vi "TDMS-File Viewer.vi"(4 "error in (no error)":errorcluster, 7 "file path":path) -> (0 "error out":errorcluster, 3 "file path out":path)   [LabVIEW 2010]
doc: "Opens the .tdms file specified in the <B>file path</B> input and presents the file data in the TDMS File Viewer dialog box."
uses:
  <vilib>/Utility/tdmsutil.llb/fileViewerConfigData.ctl
  <vilib>/Utility/tdmsutil.llb/TDMSFileViewerLocalizedText.vi
  Instance           1 26Saved   TDMS - File Viewer .vi
panel:
  in  "Help":bool
  in  "Status":string
  in  "Quit":bool
  in  "Settings...":bool
  in  "Properties / Values / Graph":T1(tab)
  in  "Properties":i32(listbox)
  in  "Raw data values":i32(listbox)
  out "Waveform Graph":waveform(dbl)[](graph)
  in  "File contents":string(tree)
  # "Displaying values 1..1000"
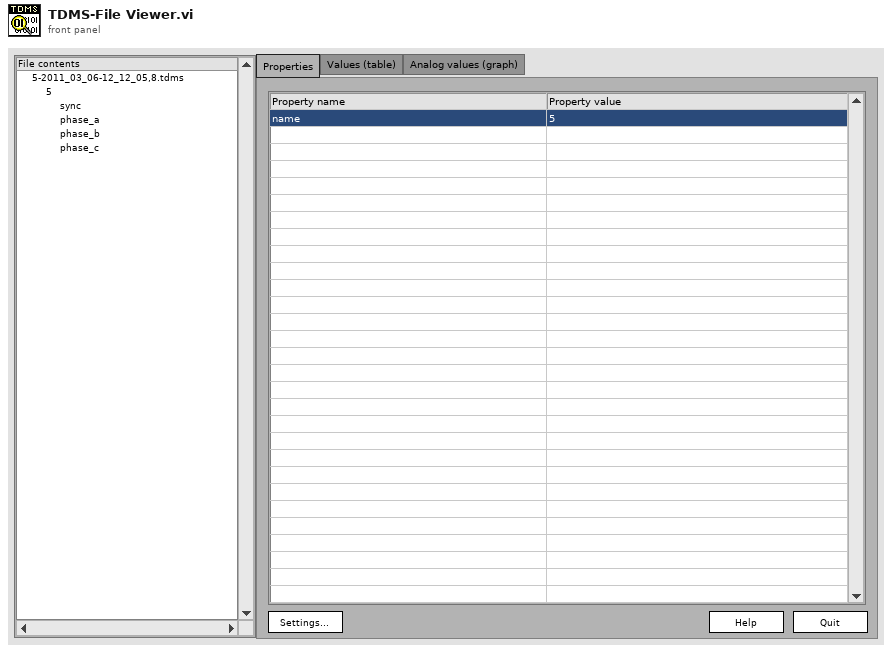
[diagram p1: front panel]
types:
  T1 = enum32{"Properties", "Values (table)", "Analog values (graph)"}
  T2 = enum16{"open", "open or create", "create or replace", "create", "open (read-only)"}
  T3 = typedef "fileViewerConfigData.ctl" = cluster{"Show all (table)":bool, "Show all (graph)":bool, "limit (table)":u64, "limit (graph)":u64, "no show":bool, "start (table)":u64, "start (graph)":u64}
  T4 = cluster{"Tree":refnum<vi>, "Tab Control":refnum<vi>, "property list":refnum<vi>, "raw data list":refnum<vi>, "Waveform Graph":refnum<vi>, "Ok":refnum<vi>, "Ok 2":refnum<vi>, "Ok 3":refnum<vi>, "Ok 4":refnum<vi>}
  T5 = typedef "LVRectTypeDef.ctl" = cluster{"left":i16, "top":i16, "right":i16, "bottom":i16}
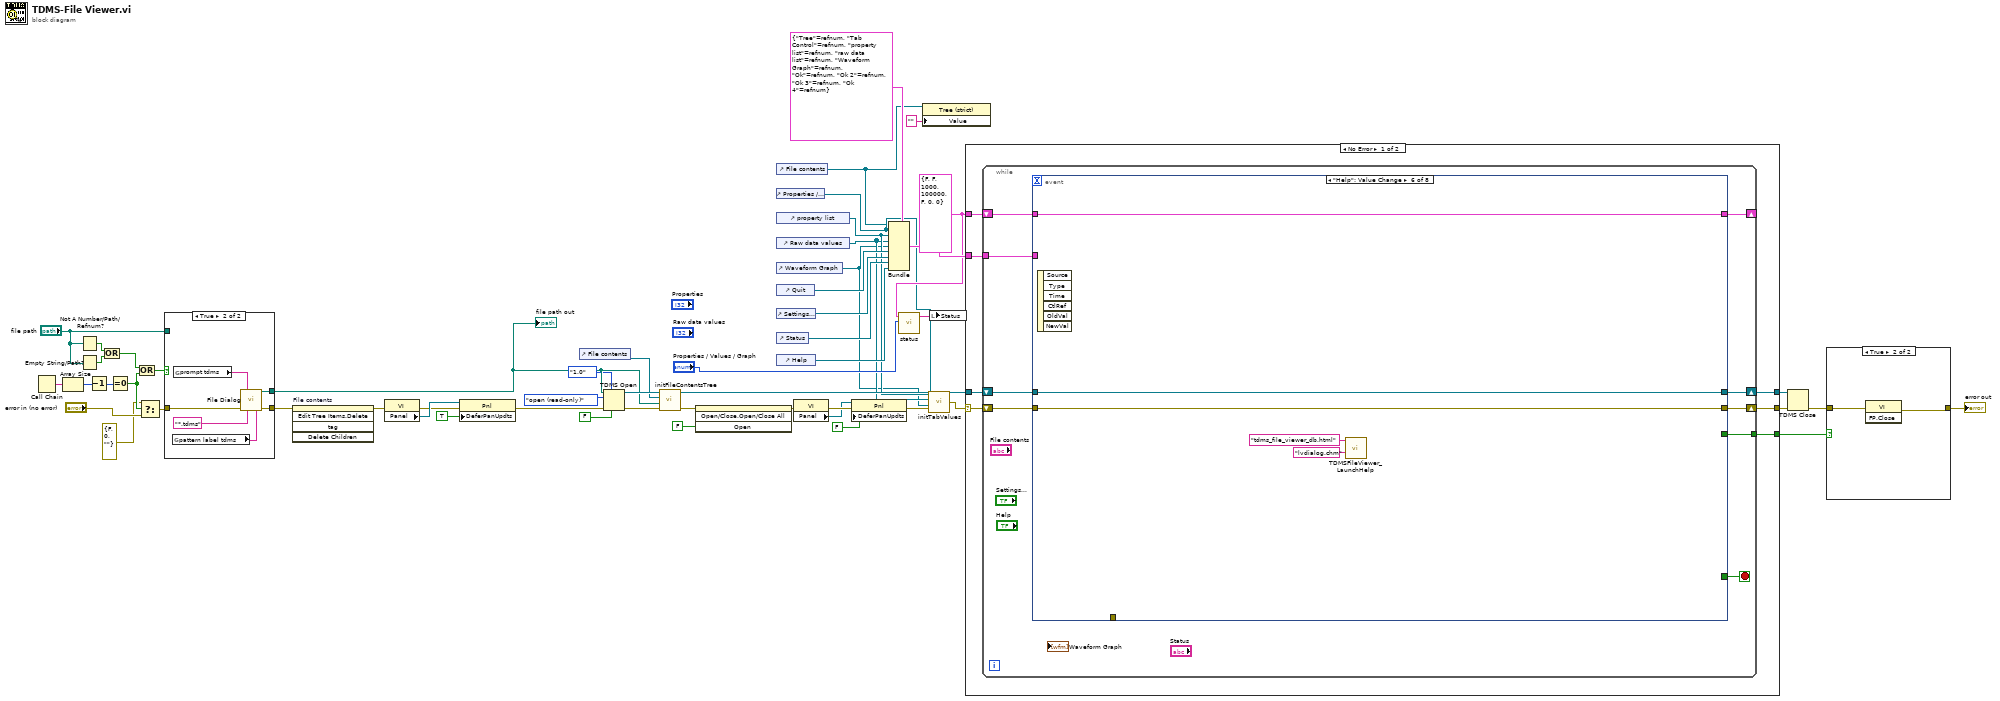
[diagram p0: block diagram]
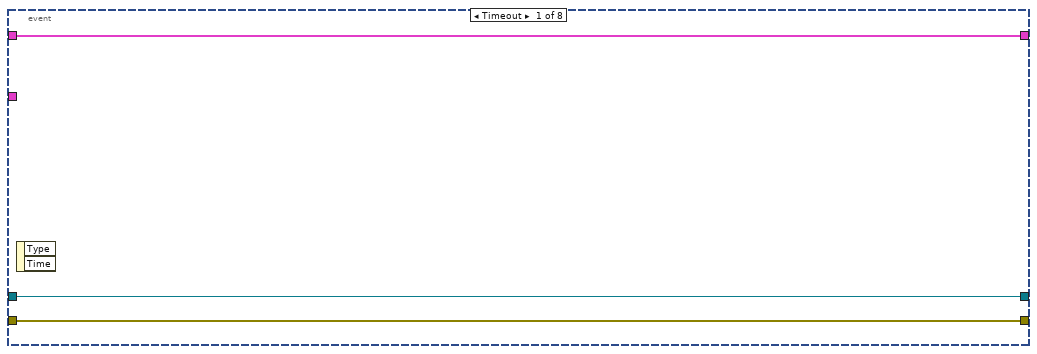
[diagram p3: hidden frame]
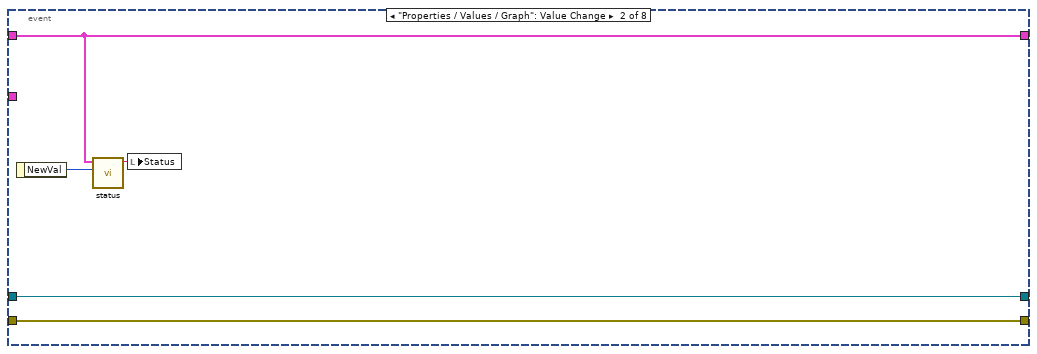
[diagram p4: hidden frame]
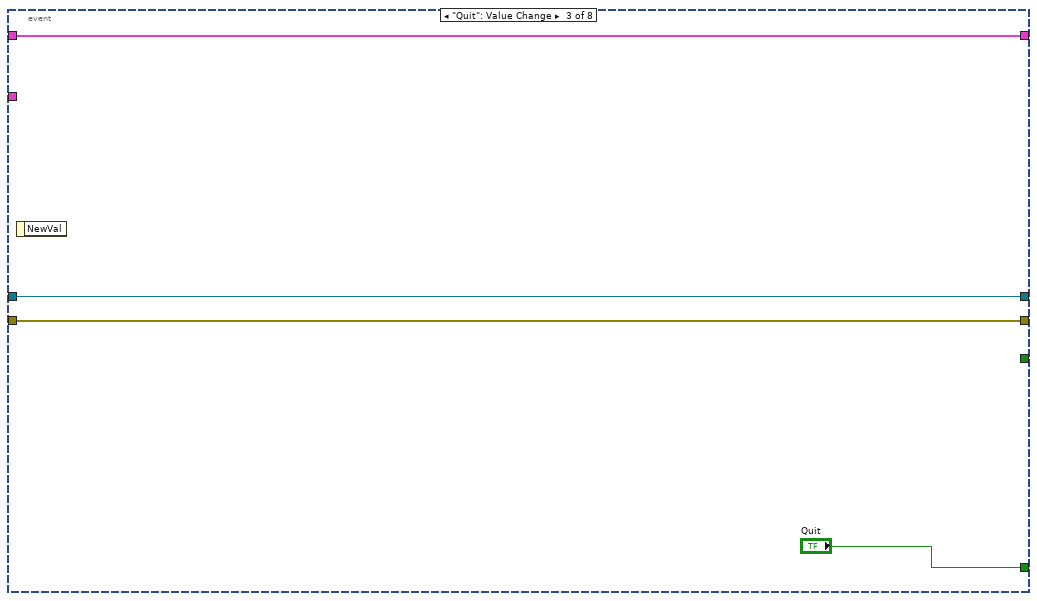
[diagram p5: hidden frame]
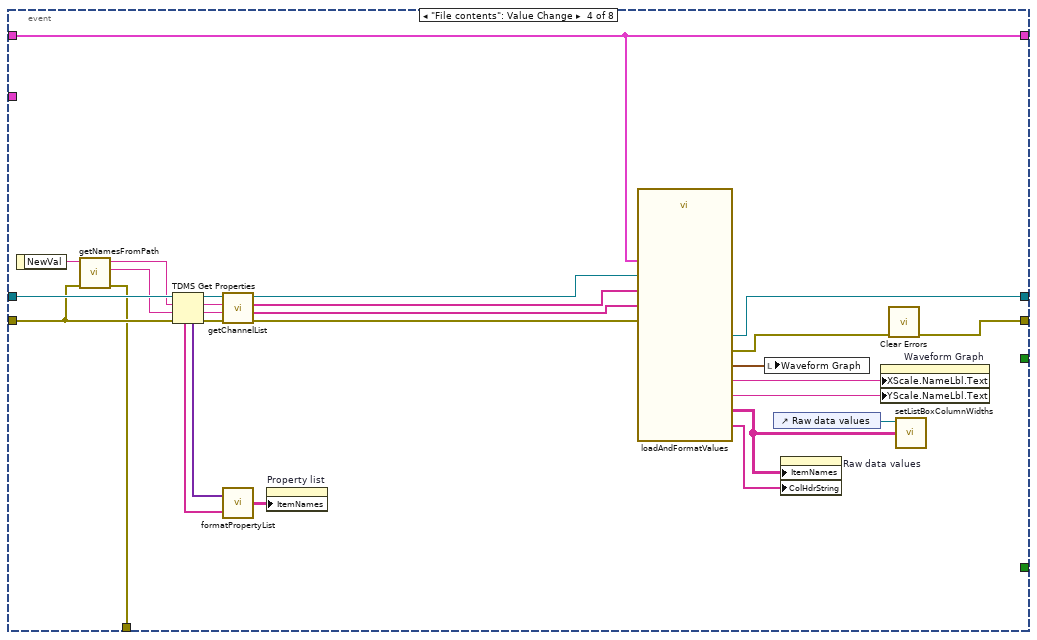
[diagram p6: hidden frame]
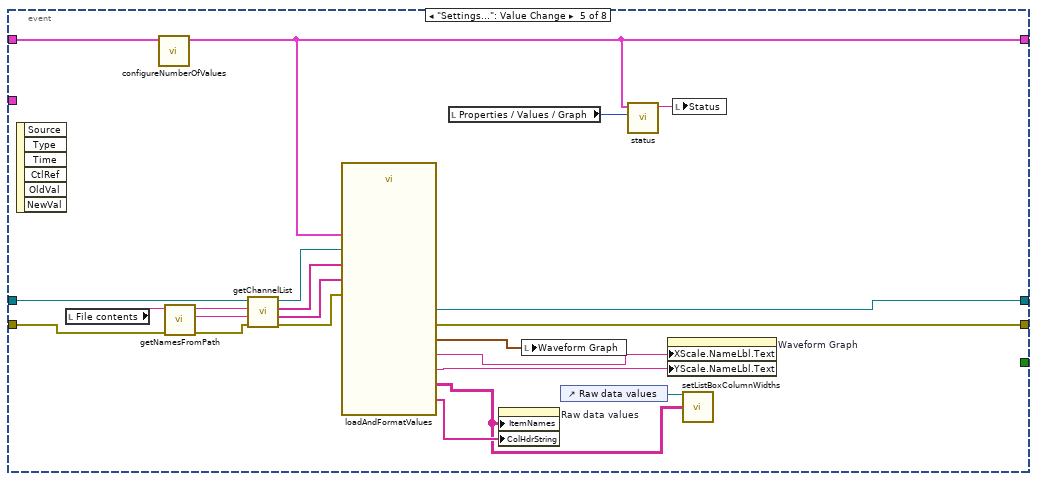
[diagram p7: hidden frame]
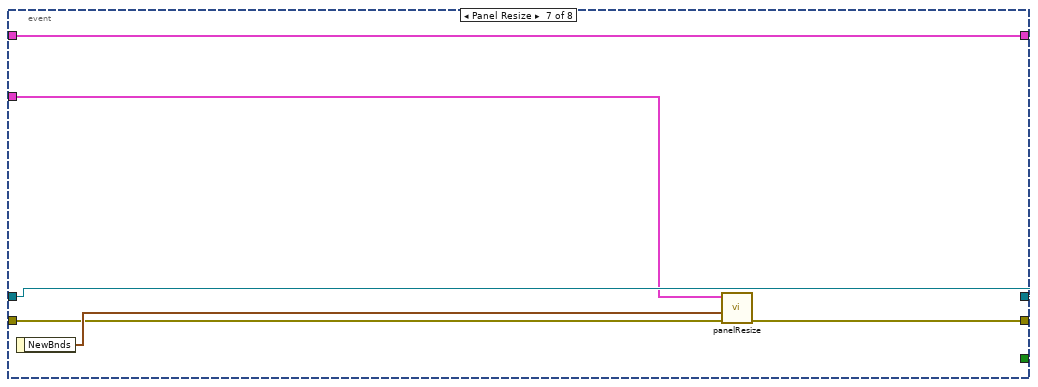
[diagram p8: hidden frame]
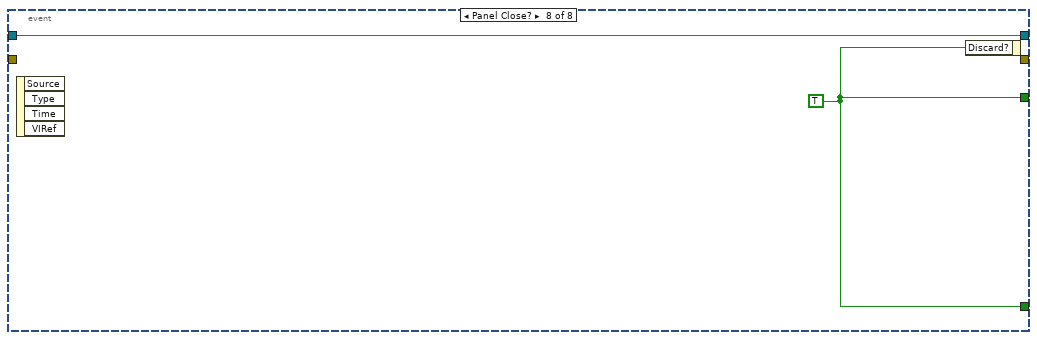
[diagram p9: hidden frame]
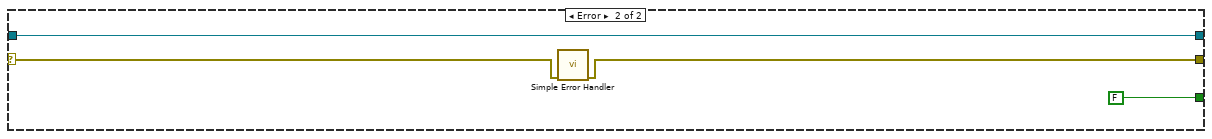
[diagram p10: hidden frame]
diagram:
  w20 = T3 {"Show all (table)"=FALSE, "Show all (graph)"=FALSE, "limit (table)"=1000, "limit (graph)"=100000, "no show"=FALSE, "start (table)"=0, "start (graph)"=0} ("TDMS File Viewer Configuration")
  n1 = Call Chain() -> (call chain=w35:string[])
  n2 = Array Size(array=w35) -> (size(s)=w33:i32)
  n3 = Not A Number/Path/Refnum?(number/path/refnum="file path") -> (NaN/Path/Refnum?=w37:bool)
  n4 = Empty String/Path?(string/path="file path") -> (empty?=w36:bool)
  n5 = Decrement(x=w33) -> (x-1=w32:i32)
  n6 = Or(x=w37, y=w36) -> (x .or. y?=w34:bool)
  n7 = Equal To 0?(x=w32) -> (x = 0?=w18:bool)
  n8 = Or(x=w34, y=w18) -> (x .or. y?=w31:bool)
  n9 = Select(t=errorcluster {"status"=FALSE, "code"=0, "source"=""}, s=w18, f="error in (no error)") -> (s? t:f=w17:errorcluster)
  n10 = case shown="True" w31 {
    tunnel: [w56 w62] -> w24
    tunnel: "file path" -> [w56 _]
    tunnel: [w55 w60] -> w23
    tunnel: w17 -> [w55 w59]
    frame False {
    }
    frame True {
      n11 = global read "TDMSFileViewerLocalizedText.vi" "pattern label tdms"() -> (w57:string)
      n12 = global read "TDMSFileViewerLocalizedText.vi" "prompt tdms"() -> (w58:string)
      n13 = call "File Dialog"("prompt"=w58, "error in"=w59, "pattern (all files)"="*.tdms", "pattern label"=w57) -> ("selected path"=w62:path, "error out"=w60:errorcluster)  [unwired: 3 in, 7 out]
    }
  }
  "file path out" <- w24
  n14 = invoke on="File contents" class="Tree (strict)" method="Edit Tree Items.Delete"(error in=w23) -> (error out=w45:errorcluster)  [unwired: 4 in, 4 out]
  n15 = property class="VI"(error in=w45) -> (error out=w46:errorcluster, "Panel"=w47:refnum<vi>)  [unwired: 1 in, 1 out]
  n16 = property class="Pnl"(reference=w47, error in=w46, "DeferPanUpdts"=TRUE ("Defer Panel Updates")) -> (error out=w49:errorcluster)  [unwired: 1 out]
  n17 = control-ref of="File contents"() -> (w25:refnum<vi>)
  n18 = TDMS Open(6:FALSE ("disable buffering (T)"), 7:enum16{"1.0", "2.0"}."1.0" ("file format version (2.0)"), 8:w49, 10:T2."open (read-only)" ("operation"), 11:w24) -> (0:w54:errorcluster, 3:w53:refnum<k34>)  [unwired: 1 in]
  n19 = call <vilib>:"initFileContentsTree.vi"("error in (no error)"=w54, "file path"=w24, "Tree Refnum"=w25, "tdms file"=w53) -> ("error out"=w41:errorcluster, "tdms file out"=w52:refnum<k34>)  [unwired: 2 out]
  n20 = invoke on="File contents" class="Tree (strict)" method="Open/Close.Open/Close All"(error in=w41, "Open"=FALSE ("Open?")) -> (error out=w40:errorcluster)  [unwired: 2 in, 3 out]
  n21 = control-ref of="File contents"() -> (w2:refnum<vi>)
  n22 = control-ref of="Properties / Values / Graph"() -> (w3:refnum<vi>)
  n23 = control-ref of="property list"() -> (w6:refnum<vi>)
  n24 = control-ref of="Raw data values"() -> (w5:refnum<vi>)
  n25 = control-ref of="Waveform Graph"() -> (w4:refnum<vi>)
  n26 = control-ref of="Quit"() -> (w29:refnum<vi>)
  n27 = control-ref of="Settings..."() -> (w27:refnum<vi>)
  n28 = control-ref of="Status"() -> (w22:refnum<vi>)
  n29 = control-ref of="Help"() -> (w9:refnum<vi>)
  n30 = property class="VI"(error in=w40) -> (error out=w43:errorcluster, "Panel"=w42:refnum<vi>)  [unwired: 1 in, 1 out]
  n31 = property class="Pnl"(reference=w42, error in=w43, "DeferPanUpdts"=FALSE ("Defer Panel Updates")) -> (error out=w8:errorcluster)  [unwired: 1 out]
  n32 = Bundle(cluster=T4 {"Tree"=refnum, "Tab Control"=refnum, "property list"=refnum, "raw data list"=refnum, "Waveform Graph"=refnum, "Ok"=refnum, "Ok 2"=refnum, "Ok 3"=refnum, "Ok 4"=refnum} ("control refs"), "Tree"=w2, "Tab Control"=w3, "property list"=w6, "raw data list"=w5, "Waveform Graph"=w4, "Ok"=w29, "Ok 2"=w27, "Ok 3"=w22, "Ok 4"=w9) -> (w30:T4)
  n33 = call <vilib>:"status.vi"("tab sheet"="Properties / Values / Graph", "TDMS File Viewer Configuration"=w20) -> ("status"=w21:string)  [unwired: 5 out]
  n34 = property class="Tree (strict)"(reference=w2, "Value"="") -> ()  [unwired: 1 in, 2 out]
  n35 = call <vilib>:"initTabValues.vi"("properties"=w6, "Values"=w5, "waveform"=w4, "error in"=w8, "Properties / Values / Graph"=w3) -> ("error out"=w7:errorcluster)
  n36 = local write "Status"(w21) -> ()
  n37 = case shown="No Error" w7 {
    selector: w7 -> [w64 w155]
    tunnel: w52 -> [w69 w156]
    tunnel: [w68 w156] -> w51
    tunnel: [w67 w154] -> w50
    tunnel: w30 -> [w66 _]
    tunnel: w20 -> [w65 _]
    tunnel: [w63 FALSE] -> w14
    frame No Error {
      n38 = while {
        shift-right: [w76] -> w67
        shift-left: w64 -> [w77]
        shift-right: [w75] -> w68
        shift-left: w69 -> [w78]
        tunnel: w66 -> [w73]
        shift-right: [w71] -> _
        shift-left: w65 -> [w72]
        tunnel: [w70] -> w63
        stop <- w74 stop-if-true
        n39 = event shown="[5] \"Help\": Value Change" {
          selector: _ -> [_ _ _ _ _ _ _ _]
          dyn-events: _ -> [_ _ _ _ _ _ _ _]
          timeout: _ -> [_ _ _ _ _ _ _ _]
          tunnel: w78 -> [w80 w85 w89 w117 w128 w143 w150 w152]
          tunnel: w77 -> [w81 w86 w88 w109 w136 w142 w147 _]
          tunnel: [w81 w86 w88 w104 w137 w142 w146 _] -> w76
          tunnel: [w80 w85 w89 w116 w138 w143 w150 w152] -> w75
          tunnel: [_ _ "Quit" _ _ _ _ w151] -> w74
          tunnel: [_ _ _ w108 _ _ _ _] -> _
          tunnel: w73 -> [_ _ _ _ _ _ w148 _]
          tunnel: w72 -> [w79 w82 w87 w97 w139 w144 w145 _]
          tunnel: [w79 w82 w87 w97 w118 w144 w145 _] -> w71
          tunnel: [_ _ _ _ _ _ _ w151] -> w70
          event Timeout {
            n40 = event-data() -> ()  [unwired: 3 out]
          }
          event "Properties / Values / Graph": Value Change {
            n41 = event-data() -> ("NewVal"=w84:T1)  [unwired: 1 out]
            n42 = call <vilib>:"status.vi"("tab sheet"=w84, "TDMS File Viewer Configuration"=w82) -> ("status"=w83:string)  [unwired: 5 out]
            n43 = local write "Status"(w83) -> ()
          }
          event "Quit": Value Change {
            n44 = event-data() -> ()  [unwired: 2 out]
          }
          event "File contents": Value Change {
            n45 = event-data() -> ("NewVal"=w111:string)  [unwired: 1 out]
            n46 = call <vilib>:"getNamesFromPath.vi"("error in (no error)"=w109, "tree path"=w111) -> ("error out"=w108:errorcluster, "channel"=w114:string, "group"=w115:string)  [unwired: 3 out]
            n47 = TDMS Get Properties(8:w109, 9:w114, 10:w115, 11:w117) -> (0:w102:errorcluster, 1:w101:string, 2:w95:string, 3:w103:refnum<k34>, 4:w112:variant[], 6:w113:string[])  [unwired: 2 out]
            n48 = call <vilib>:"getChannelList.vi"("error in (no error)"=w102, "channel names"=w101, "group name"=w95, "tdms file"=w103) -> ("error out"=w91:errorcluster, "channel names out"=w92:string[], "group names out"=w93:string[], "tdms file out"=w94:refnum<k34>)
            n49 = call <vilib>:"formatPropertyList.vi"("property names"=w113, "property values"=w112) -> ("strings"=w110:string[][])
            n50 = property on="Property list" class="MCListbox (strict)"("ItemNames"=w110) -> ()  [unwired: 2 in, 2 out]
            n51 = call <vilib>:"loadAndFormatValues.vi"("error in (no error)"=w91, "configuration"=w97, "channel names"=w92, "group names"=w93, "tdms file"=w94) -> ("error out"=w105:errorcluster, "graph y names"=w99:string, "graph x names"=w98:string, "tdms file out"=w116:refnum<k34>, "waveform values"=w96:waveform(dbl)[], "table values"=w107:string[][], "table headers"=w100:string[])
            n52 = local write "Waveform Graph"(w96) -> ()
            n53 = control-ref of="Raw data values"() -> (w106:refnum<vi>)
            n54 = property on="Raw data values" class="MCListbox (strict)"("ItemNames"=w107, "ColHdrString"=w100) -> ()  [unwired: 2 in, 2 out]
            n55 = property on="Waveform Graph" class="WFGraph (strict)"("XScale.NameLbl.Text"=w98, "YScale.NameLbl.Text"=w99) -> ()  [unwired: 2 in, 2 out]
            n56 = call <vilib>:"Clear Errors.vi"("error in (no error)"=w105) -> ("error out"=w104:errorcluster)  [unwired: 6 out]
            n57 = call <vilib>:"setListBoxColumnWidths.vi"("table data"=w107, "MCListbox Refnum"=w106) -> ()  [unwired: 1 out]
          }
          event "Settings...": Value Change {
            n58 = event-data() -> ()  [unwired: 7 out]
            n59 = local read "File contents"() -> (w129:string)
            n60 = call <vilib>:"configureNumberOfValues.vi"("TDMS File Viewer Configuration"=w139) -> ("TDMS File Viewer Configuration Out"=w118:T3)  [unwired: 10 out]
            n61 = call <vilib>:"getNamesFromPath.vi"("error in (no error)"=w136, "tree path"=w129) -> ("error out"=w127:errorcluster, "channel"=w125:string, "group"=w126:string)  [unwired: 3 out]
            n62 = call <vilib>:"getChannelList.vi"("error in (no error)"=w127, "channel names"=w125, "group name"=w126, "tdms file"=w128) -> ("error out"=w124:errorcluster, "channel names out"=w121:string[], "group names out"=w122:string[], "tdms file out"=w123:refnum<k34>)
            n63 = call <vilib>:"loadAndFormatValues.vi"("error in (no error)"=w124, "configuration"=w118, "channel names"=w121, "group names"=w122, "tdms file"=w123) -> ("error out"=w137:errorcluster, "graph y names"=w131:string, "graph x names"=w130:string, "tdms file out"=w138:refnum<k34>, "waveform values"=w135:waveform(dbl)[], "table values"=w132:string[][], "table headers"=w134:string[])
            n64 = local read "Properties / Values / Graph"() -> (w119:T1)
            n65 = property on="Raw data values" class="MCListbox (strict)"("ItemNames"=w132, "ColHdrString"=w134) -> ()  [unwired: 2 in, 2 out]
            n66 = local write "Waveform Graph"(w135) -> ()
            n67 = control-ref of="Raw data values"() -> (w133:refnum<vi>)
            n68 = call <vilib>:"status.vi"("tab sheet"=w119, "TDMS File Viewer Configuration"=w118) -> ("status"=w120:string)  [unwired: 5 out]
            n69 = property on="Waveform Graph" class="WFGraph (strict)"("XScale.NameLbl.Text"=w130, "YScale.NameLbl.Text"=w131) -> ()  [unwired: 2 in, 2 out]
            n70 = local write "Status"(w120) -> ()
            n71 = call <vilib>:"setListBoxColumnWidths.vi"("table data"=w132, "MCListbox Refnum"=w133) -> ()  [unwired: 1 out]
          }
          event "Help": Value Change {
            n72 = event-data() -> ()  [unwired: 7 out]
            n73 = call <vilib>:"TDMSFileViewer_LaunchHelp.vi"("CHM or HLP filename (lvdialog.chm)"="lvdialog.chm", "HTML filename"="tdms_file_viewer_db.html") -> ()  [unwired: 1 in, 5 out]
          }
          event Panel Resize {
            n74 = event-data() -> ("NewBnds"=w149:T5)  [unwired: 1 out]
            n75 = call <vilib>:"panelResize.vi"("error in (no error)"=w147, "NewBnds"=w149, "control refs"=w148) -> ("error out"=w146:errorcluster)  [unwired: 4 in]
          }
          event Panel Close? {
            w151 = TRUE
            n76 = event-data() -> ()  [unwired: 5 out]
            n77 = event-data("Discard?"=w151) -> ()  [unwired: 1 in, 1 out]
          }
        }
      }
    }
    frame Error {
      n78 = call <vilib>:"Simple Error Handler.vi"("error in (no error)"=w155) -> ("error out"=w154:errorcluster)  [unwired: 1 in, 7 out]
    }
  }
  n79 = TDMS Close(8:w50, 11:w51) -> (0:w13:errorcluster)  [unwired: 1 out]
  n80 = case shown="True" w14 {
    tunnel: w13 -> [w157 w159]
    tunnel: [w157 w158] -> w12
    frame False {
    }
    frame True {
      n81 = invoke class="VI" method="FP.Close"(error in=w159) -> (error out=w158:errorcluster)  [unwired: 2 in, 2 out]
    }
  }
  "error out" <- w12
